vi "Set Valid Index Range.vi"(8 "error in":errorcluster, 10 "Valid Index Range":cluster{"Lower":u16, "Upper":u16}={"Lower"=6656, "Upper"=7167} {"Upper" format="%.0x"; "Lower" format="%.0x"}, 11 "PDO Mapping in":refnum<class "PDO Mapping.lvclass">) -> (0 "error out":errorcluster, 3 "PDO Mapping out":refnum<class "PDO Mapping.lvclass">)   [LabVIEW 2020, in "CANopen.lvlib" / "PDO Mapping.lvclass"]
uses:
  PDO Mapping.lvclass
  PDO Mapping.lvclass/PDO Mapping.ctl
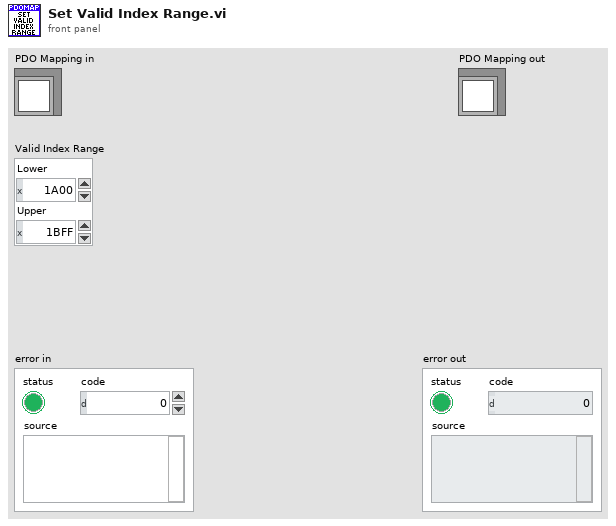
[diagram p1: front panel]
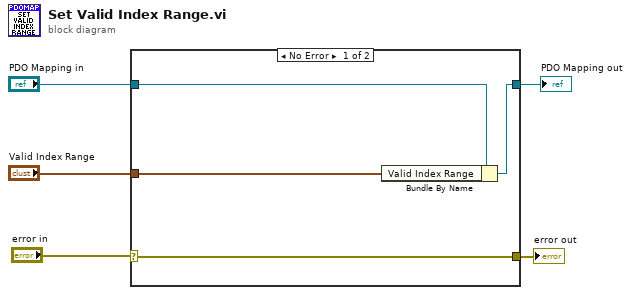
[diagram p0: block diagram]
diagram:
  n1 = case shown="No Error" "error in" {
    selector: "error in" -> [w9 w10]
    tunnel: [w9 w10] -> w2
    tunnel: [w7 w11] -> w4
    tunnel: "PDO Mapping in" -> [w8 w11]
    tunnel: "Valid Index Range" -> [w6 _]
    frame No Error {
      n2 = Bundle By Name(cluster=w8, "Valid Index Range"=w6) -> (w7:refnum<class "PDO Mapping.lvclass">)
    }
    frame Error {
    }
  }
  "error out" <- w2
  "PDO Mapping out" <- w4
